vi "ForceAnnotationMan.vi"(4 "EnReturnForce":bool, 5 "EnFullAngle":bool, 6 "SpectConfig":T4, 7 "FirstTouch":T3={"FirstPeakforce"=0.2, "F_LengthView"=0, "A_LengthView "=0} {"FirstPeakforce" format="%#_13g"}, 8 "ShowName":cluster{"ShowArrow":bool, "Alias":bool}, 9 "Test Name":string(combo)="WDW", 10 "Graph Up":refnum<vi>, 11 "Graph Down":refnum<vi>) -> (0 "MaxForceUp":T2, 1 "Result Up":T1, 2 "Result Down":T1, 3 "MaxForceDown":T2)   [LabVIEW 2017]
uses:
  <vilib>/Utility/miscctls.llb/LVAnnotationListTypeDef.ctl
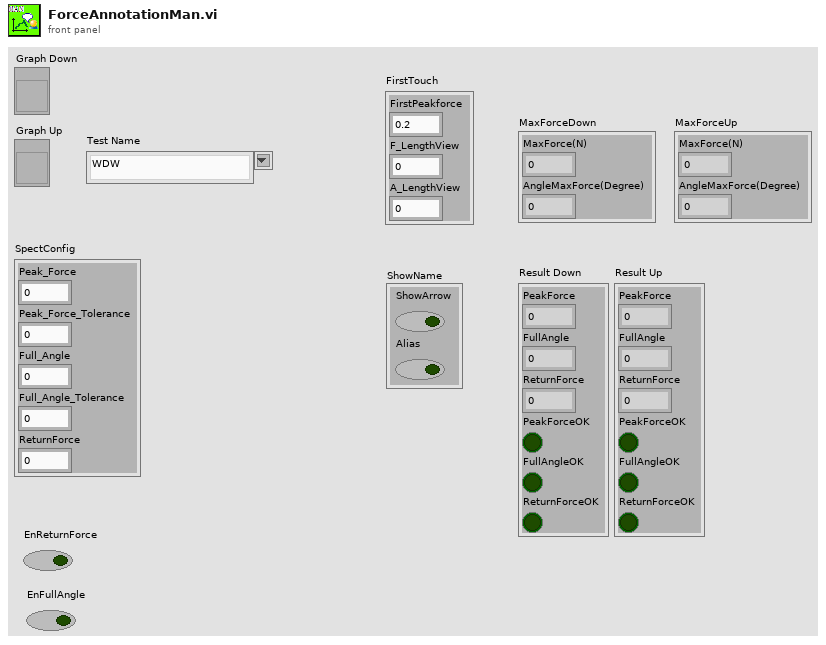
[diagram p1: front panel]
types:
  T1 = cluster{"PeakForce":dbl, "FullAngle":dbl, "ReturnForce":dbl, "PeakForceOK":bool, "FullAngleOK":bool, "ReturnForceOK":bool}
  T2 = cluster{"MaxForce(N)":dbl, "AngleMaxForce(Degree)":dbl}
  T3 = cluster{"FirstPeakforce":dbl, "F_LengthView":i32, "A_LengthView ":i32}
  T4 = cluster{"Peak_Force":dbl, "Peak_Force_Tolerance":dbl, "Full_Angle":dbl, "Full_Angle_Tolerance":dbl, "ReturnForce":dbl}
  T5 = cluster{"FirstForce":dbl, "LengthView":i32, "Name":string}
  T6 = typedef "LVAnnotationListTypeDef.ctl" = cluster{"Name":string, "Color":u32, "Style":u8, "Point Style":u8, "Name Visible":bool, "Allow Drag":bool, "Annotation Mode":u32, "Plot":i32, "Index":i32, "Position":cluster{"X":dbl, "Y":dbl}, "X Scale":u32, "Y Scale":u32, "Show Arrow":bool, "Lock Name":bool, "Plot Area":i32, "Label Offset":cluster{"X":dbl, "Y":dbl}}[]
  T7 = cluster{"Annotation List[0]":cluster{"Name":string, "Color":u32, "Style":u8, "Point Style":u8, "Name Visible":bool, "Allow Drag":bool, "Annotation Mode":u32, "Plot":i32, "Index":i32, "Position":cluster{"X":dbl, "Y":dbl}, "X Scale":u32, "Y Scale":u32, "Show Arrow":bool, "Lock Name":bool, "Plot Area":i32, "Label Offset":cluster{"X":dbl, "Y":dbl}}, "Annotation List[1]":cluster{"Name":string, "Color":u32, "Style":u8, "Point Style":u8, "Name Visible":bool, "Allow Drag":bool, "Annotation Mode":u32, "Plot":i32, "Index":i32, "Position":cluster{"X":dbl, "Y":dbl}, "X Scale":u32, "Y Scale":u32, "Show Arrow":bool, "Lock Name":bool, "Plot Area":i32, "Label Offset":cluster{"X":dbl, "Y":dbl}}, "Annotation List[2]":cluster{"Name":string, "Color":u32, "Style":u8, "Point Style":u8, "Name Visible":bool, "Allow Drag":bool, "Annotation Mode":u32, "Plot":i32, "Index":i32, "Position":cluster{"X":dbl, "Y":dbl}, "X Scale":u32, "Y Scale":u32, "Show Arrow":bool, "Lock Name":bool, "Plot Area":i32, "Label Offset":cluster{"X":dbl, "Y":dbl}}, "Annotation List[3]":cluster{"Name":string, "Color":u32, "Style":u8, "Point Style":u8, "Name Visible":bool, "Allow Drag":bool, "Annotation Mode":u32, "Plot":i32, "Index":i32, "Position":cluster{"X":dbl, "Y":dbl}, "X Scale":u32, "Y Scale":u32, "Show Arrow":bool, "Lock Name":bool, "Plot Area":i32, "Label Offset":cluster{"X":dbl, "Y":dbl}}, "Annotation List[4]":cluster{"Name":string, "Color":u32, "Style":u8, "Point Style":u8, "Name Visible":bool, "Allow Drag":bool, "Annotation Mode":u32, "Plot":i32, "Index":i32, "Position":cluster{"X":dbl, "Y":dbl}, "X Scale":u32, "Y Scale":u32, "Show Arrow":bool, "Lock Name":bool, "Plot Area":i32, "Label Offset":cluster{"X":dbl, "Y":dbl}}, "Annotation List[5]":cluster{"Name":string, "Color":u32, "Style":u8, "Point Style":u8, "Name Visible":bool, "Allow Drag":bool, "Annotation Mode":u32, "Plot":i32, "Index":i32, "Position":cluster{"X":dbl, "Y":dbl}, "X Scale":u32, "Y Scale":u32, "Show Arrow":bool, "Lock Name":bool, "Plot Area":i32, "Label Offset":cluster{"X":dbl, "Y":dbl}}, "Annotation List[6]":cluster{"Name":string, "Color":u32, "Style":u8, "Point Style":u8, "Name Visible":bool, "Allow Drag":bool, "Annotation Mode":u32, "Plot":i32, "Index":i32, "Position":cluster{"X":dbl, "Y":dbl}, "X Scale":u32, "Y Scale":u32, "Show Arrow":bool, "Lock Name":bool, "Plot Area":i32, "Label Offset":cluster{"X":dbl, "Y":dbl}}, "Annotation List[7]":cluster{"Name":string, "Color":u32, "Style":u8, "Point Style":u8, "Name Visible":bool, "Allow Drag":bool, "Annotation Mode":u32, "Plot":i32, "Index":i32, "Position":cluster{"X":dbl, "Y":dbl}, "X Scale":u32, "Y Scale":u32, "Show Arrow":bool, "Lock Name":bool, "Plot Area":i32, "Label Offset":cluster{"X":dbl, "Y":dbl}}, "Annotation List[8]":cluster{"Name":string, "Color":u32, "Style":u8, "Point Style":u8, "Name Visible":bool, "Allow Drag":bool, "Annotation Mode":u32, "Plot":i32, "Index":i32, "Position":cluster{"X":dbl, "Y":dbl}, "X Scale":u32, "Y Scale":u32, "Show Arrow":bool, "Lock Name":bool, "Plot Area":i32, "Label Offset":cluster{"X":dbl, "Y":dbl}}}
  T8 = cluster{"Name":string, "Color":u32, "Style":u8, "Point Style":u8, "Name Visible":bool, "Allow Drag":bool, "Annotation Mode":u32, "Plot":i32, "Index":i32, "Position":cluster{"X":dbl, "Y":dbl}, "X Scale":u32, "Y Scale":u32, "Show Arrow":bool, "Lock Name":bool, "Plot Area":i32, "Label Offset":cluster{"X":dbl, "Y":dbl}}[]
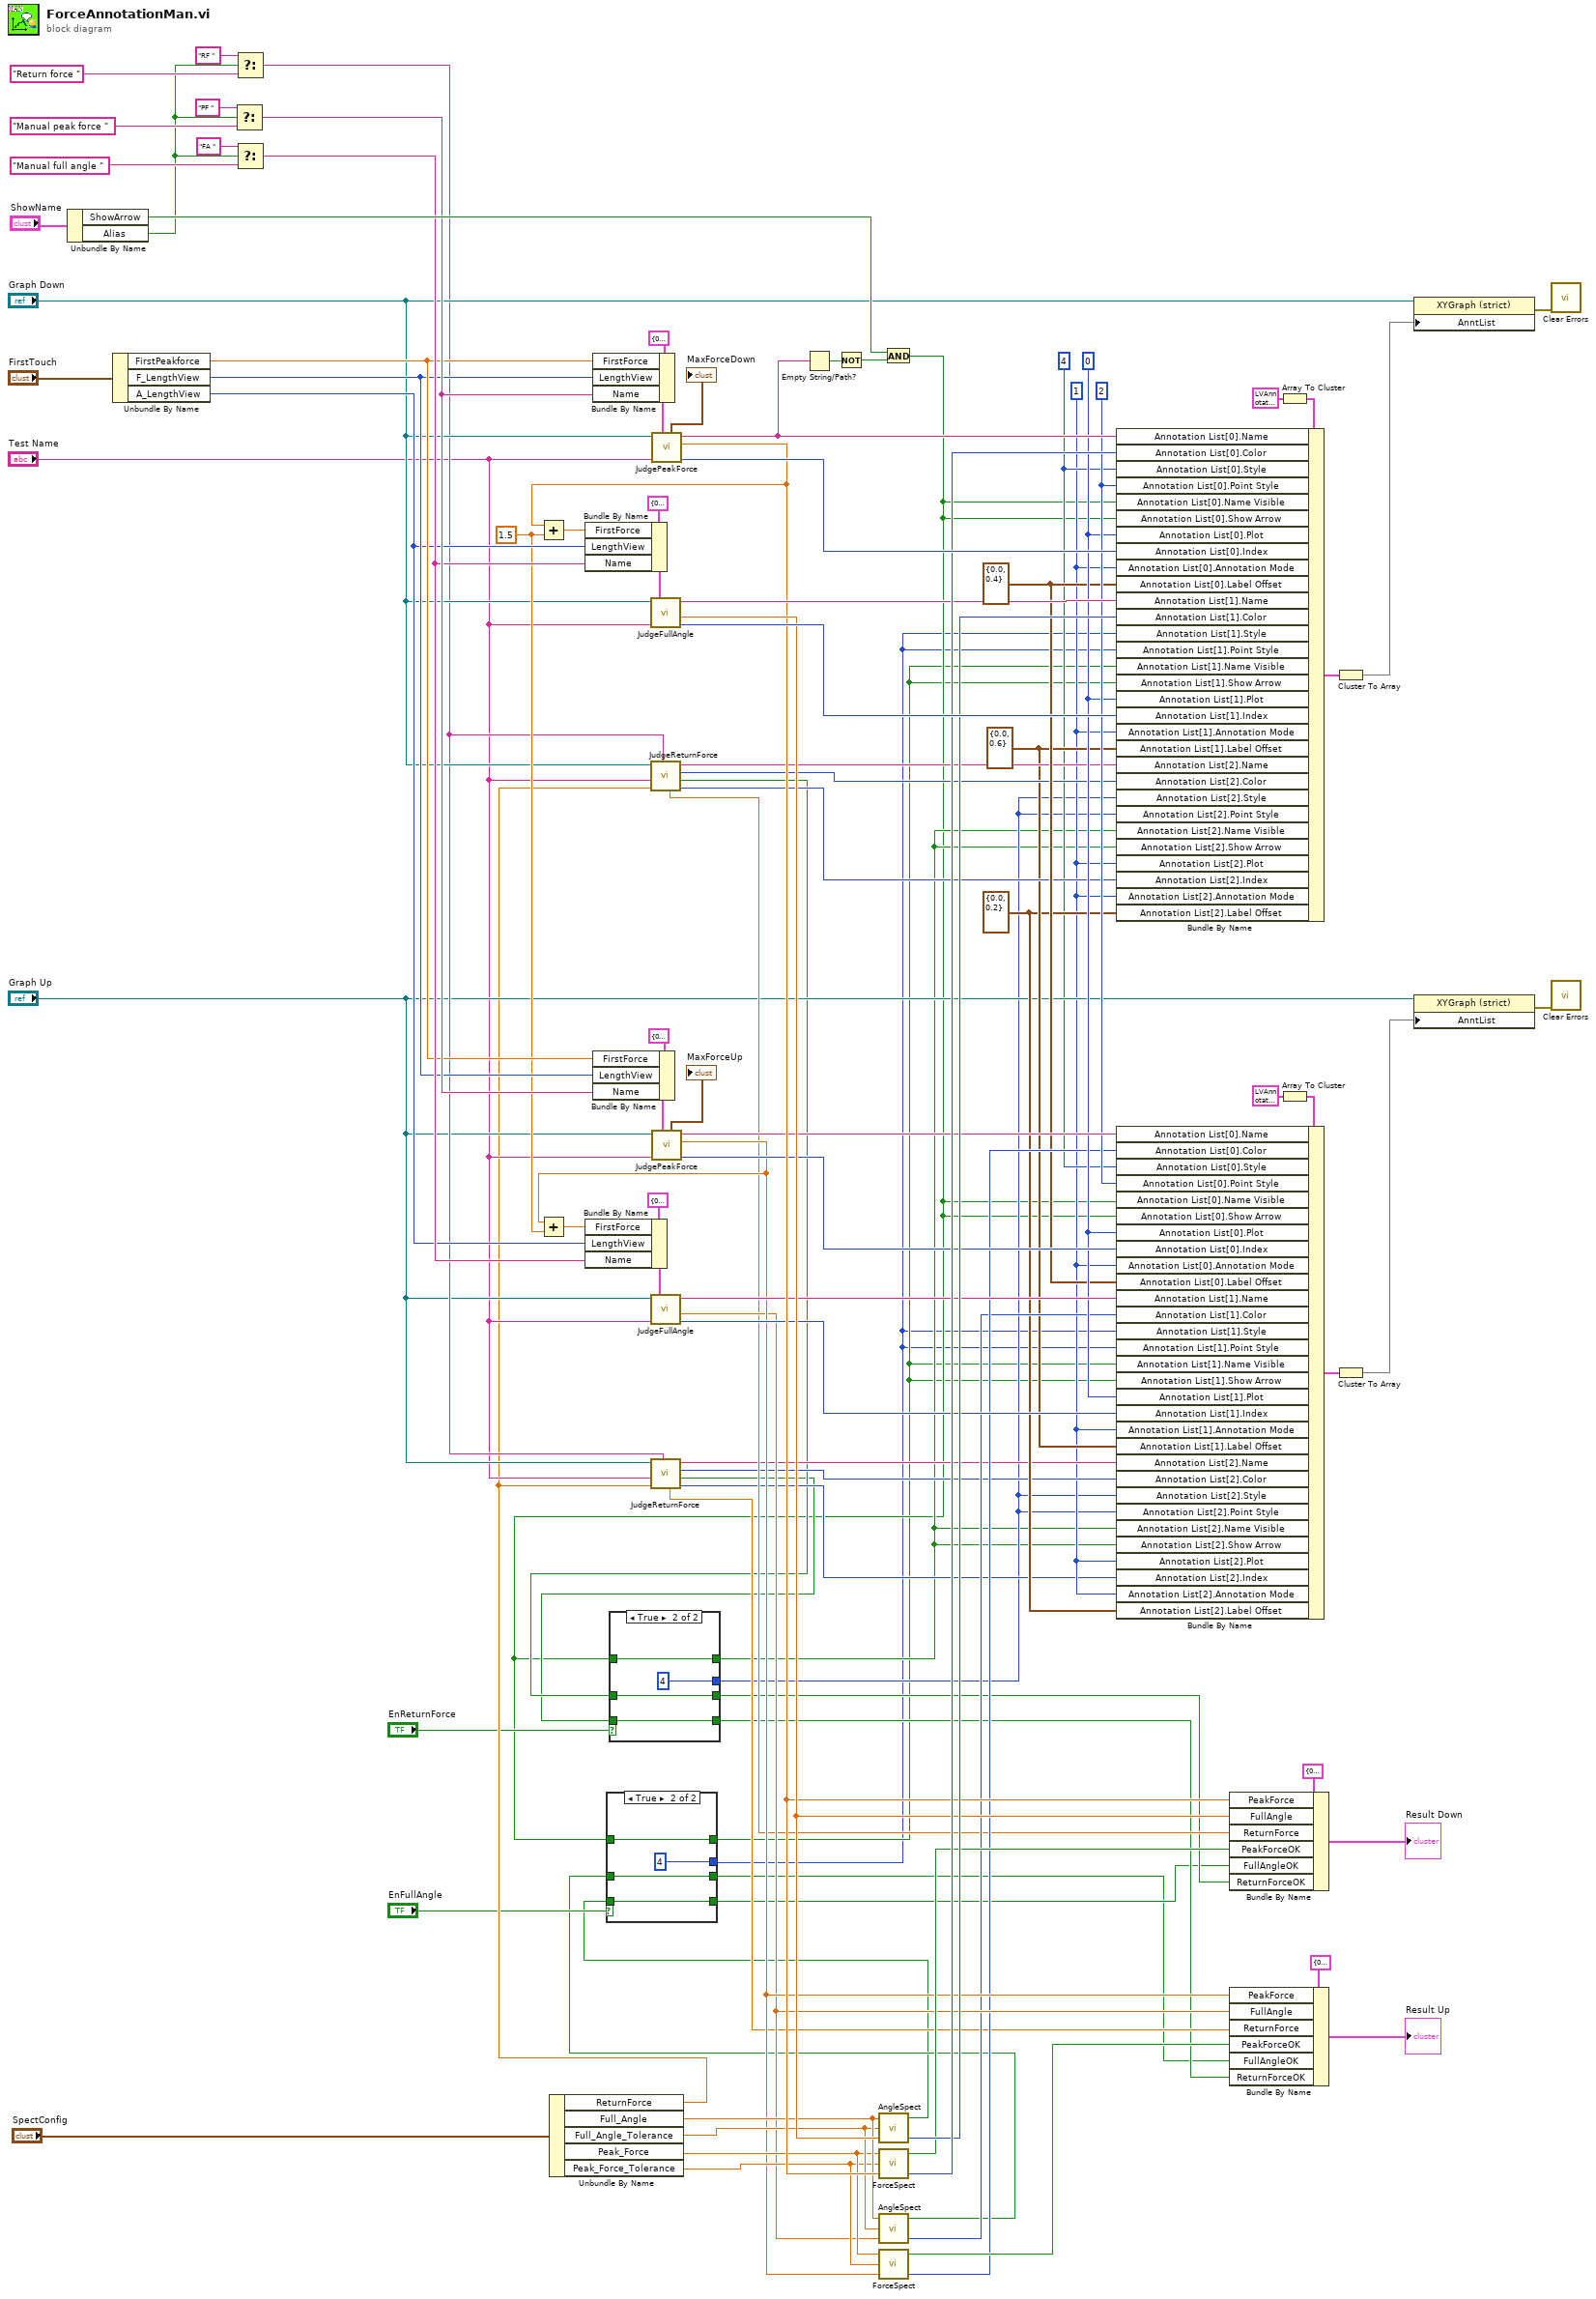
[diagram p0: block diagram]
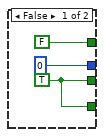
[diagram p2: hidden frame]
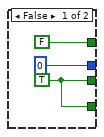
[diagram p3: hidden frame]
diagram:
  w26 = cluster{"X":dbl, "Y":dbl} {"X"=0.0, "Y"=0.2} ("Annotation List[2].Label Offset")
  w42 = 0 ("Annotation List[0].Plot")
  w38 = 1.5 ("y")
  w43 = u8 2 ("Annotation List[0].Point Style")
  w27 = cluster{"X":dbl, "Y":dbl} {"X"=0.0, "Y"=0.6} ("Annotation List[2].Label Offset")
  w39 = cluster{"X":dbl, "Y":dbl} {"X"=0.0, "Y"=0.4} ("Annotation List[0].Label Offset")
  w18 = u32 1 ("Annotation List[0].Annotation Mode")
  w19 = u8 4 ("Annotation List[0].Style")
  n1 = Unbundle By Name("ShowName") -> ("ShowArrow"=w88:bool, "Alias"=w34:bool)
  n2 = Unbundle By Name("FirstTouch") -> ("FirstPeakforce"=w58:dbl, "F_LengthView"=w57:i32, "A_LengthView"=w56:i32)
  n3 = Select(t="PF ", s=w34, f="Manual peak force " ("Name")) -> (s? t:f=w60:string)
  n4 = Select(t="RF ", s=w34, f="Return force " ("Name")) -> (s? t:f=w24:string)
  n5 = Select(t="FA ", s=w34, f="Manual full angle " ("Name")) -> (s? t:f=w59:string)
  n6 = Unbundle By Name("SpectConfig") -> ("ReturnForce"=w21:dbl, "Full_Angle"=w55:dbl, "Full_Angle_Tolerance"=w54:dbl, "Peak_Force"=w53:dbl, "Peak_Force_Tolerance"=w52:dbl)
  n7 = Bundle By Name(cluster=T5 {"FirstForce"=0.18, "LengthView"=30, "Name"="Peak Force"} ("Config"), "FirstForce"=w58, "LengthView"=w57, "Name"=w60) -> (w77:T5)
  n8 = Bundle By Name(cluster=T5 {"FirstForce"=0.18, "LengthView"=30, "Name"="Peak Force"} ("Config"), "FirstForce"=w58, "LengthView"=w57, "Name"=w60) -> (w67:T5)
  n9 = call "JudgeReturnForce.vi"("Name"=w24, "ReturnForce"=w21, "Test Name"="Test Name", "GraphDown"="Graph Down") -> ("IndexOut"=w31:i32, "Result"=w12:bool, "ColorResult"=w32:u32, "ReturnForceValue"=w33:string, "ReturnForce"=w28:dbl)  [unwired: 3 in]
  n10 = call "JudgeReturnForce.vi"("Name"=w24, "ReturnForce"=w21, "Test Name"="Test Name", "GraphDown"="Graph Up") -> ("IndexOut"=w17:i32, "Result"=w10:bool, "ColorResult"=w20:u32, "ReturnForceValue"=w25:string, "ReturnForce"=w16:dbl)  [unwired: 3 in]
  n11 = call "JudgePeakForce.vi"("Config"=w77, "Test Name"="Test Name", "XYGraph"="Graph Down") -> ("IndexOut"=w100:i32, "ForceOut"=w74:dbl, "Force Value"=w84:string, "MaxForce"=→"MaxForceDown":T2)  [unwired: 4 in, 1 out]
  n12 = Add(x=w74, y=w38) -> (x+y=w73:dbl)
  n13 = Bundle By Name(cluster=T5 {"FirstForce"=0.18, "LengthView"=30, "Name"="Peak Force"} ("Config"), "FirstForce"=w73, "LengthView"=w56, "Name"=w59) -> (w75:T5)
  n14 = call "JudgeFullAngle.vi"("Config"=w75, "Test Name"="Test Name", "XYGraph"="Graph Down") -> ("IndexOut"=w95:i32, "AngleOut"=w80:dbl, "Force Value"=w85:string)  [unwired: 5 in, 1 out]
  n15 = call "JudgePeakForce.vi"("Config"=w67, "Test Name"="Test Name", "XYGraph"="Graph Up") -> ("IndexOut"=w47:i32, "ForceOut"=w45:dbl, "Force Value"=w49:string, "MaxForce"=→"MaxForceUp":T2)  [unwired: 4 in, 1 out]
  n16 = Add(x=w45, y=w38) -> (x+y=w70:dbl)
  n17 = Bundle By Name(cluster=T5 {"FirstForce"=0.18, "LengthView"=30, "Name"="Peak Force"} ("Config"), "FirstForce"=w70, "LengthView"=w56, "Name"=w59) -> (w69:T5)
  n18 = call "JudgeFullAngle.vi"("Config"=w69, "Test Name"="Test Name", "XYGraph"="Graph Up") -> ("IndexOut"=w46:i32, "AngleOut"=w44:dbl, "Force Value"=w48:string)  [unwired: 5 in, 1 out]
  n19 = Empty String/Path?(string/path=w84) -> (empty?=w102:bool)
  n20 = Not(x=w102) -> (.not. x?=w86:bool)
  n21 = call "AngleSpect.vi"("Angle In"=w80, "Angle Tolerance"=w54, "Angle  Spect"=w55) -> ("Angle Color"=w92:u32, "Angle OK"=w6:bool)  [unwired: 1 in]
  n22 = call "ForceSpect.vi"("Force Input"=w74, "Force Tolerance"=w52, "Force  Spect"=w53) -> ("Force Color"=w93:u32, "Force OK"=w79:bool)  [unwired: 1 in]
  n23 = call "AngleSpect.vi"("Angle In"=w44, "Angle Tolerance"=w54, "Angle  Spect"=w55) -> ("Angle Color"=w40:u32, "Angle OK"=w7:bool)  [unwired: 1 in]
  n24 = call "ForceSpect.vi"("Force Input"=w45, "Force Tolerance"=w52, "Force  Spect"=w53) -> ("Force Color"=w41:u32, "Force OK"=w50:bool)  [unwired: 1 in]
  n25 = And(x=w88, y=w86) -> (x .and. y?=w3:bool)
  n26 = case shown="True" "EnFullAngle" {
    tunnel: [0 4] -> w1
    tunnel: [FALSE w108] -> w2
    tunnel: w3 -> [_ w108]
    tunnel: w7 -> [_ w107]
    tunnel: [w103 w107] -> w4
    tunnel: w6 -> [_ w106]
    tunnel: [w103 w106] -> w5
    frame False {
      w103 = TRUE ("Result")
    }
    frame True {
    }
  }
  n27 = case shown="True" "EnReturnForce" {
    tunnel: [0 4] -> w15
    tunnel: [FALSE w115] -> w14
    tunnel: w3 -> [_ w115]
    tunnel: w12 -> [_ w114]
    tunnel: [w110 w114] -> w11
    tunnel: w10 -> [_ w113]
    tunnel: [w110 w113] -> w9
    frame False {
      w110 = TRUE ("Result")
    }
    frame True {
    }
  }
  n28 = Bundle By Name(cluster=T1 {"PeakForce"=0.0, "FullAngle"=0.0, "ReturnForce"=0.0, "PeakForceOK"=FALSE, "FullAngleOK"=FALSE, "ReturnForceOK"=FALSE} ("Result Down"), "PeakForce"=w74, "FullAngle"=w80, "ReturnForce"=w28, "PeakForceOK"=w79, "FullAngleOK"=w5, "ReturnForceOK"=w11) -> (→"Result Down":T1)
  n29 = Bundle By Name(cluster=T1 {"PeakForce"=0.0, "FullAngle"=0.0, "ReturnForce"=0.0, "PeakForceOK"=FALSE, "FullAngleOK"=FALSE, "ReturnForceOK"=FALSE} ("Result Down"), "PeakForce"=w45, "FullAngle"=w44, "ReturnForce"=w16, "PeakForceOK"=w50, "FullAngleOK"=w4, "ReturnForceOK"=w9) -> (→"Result Up":T1)
  n30 = Array To Cluster(array=T6 [{"Name"="", "Color"=0, "Style"=0, "Point Style"=0, "Name Visible"=FALSE, "Allow Drag"=FALSE, "Annotation Mode"=0, "Plot"=0, "Index"=0, "Position"={"X"=0.0, "Y"=0.0}, "X Scale"=0, "Y Scale"=0, "Show Arrow"=FALSE, "Lock Name"=FALSE, "Plot Area"=0, "Label Offset"={"X"=0.0, "Y"=0.0}}] ("Annotation List")) -> (cluster=w97:T7)
  n31 = Bundle By Name(cluster=w97, "Annotation List[0].Name"=w84, "Annotation List[0].Color"=w93, "Annotation List[0].Style"=w19, "Annotation List[0].Point Style"=w43, "Annotation List[0].Name Visible"=w3, "Annotation List[0].Show Arrow"=w3, "Annotation List[0].Plot"=w42, "Annotation List[0].Index"=w100, "Annotation List[0].Annotation Mode"=w18, "Annotation List[0].Label Offset"=w39, "Annotation List[1].Name"=w85, "Annotation List[1].Color"=w92, "Annotation List[1].Style"=w1, "Annotation List[1].Point Style"=w1, "Annotation List[1].Name Visible"=w2, "Annotation List[1].Show Arrow"=w2, "Annotation List[1].Plot"=w42, "Annotation List[1].Index"=w95, "Annotation List[1].Annotation Mode"=w18, "Annotation List[1].Label Offset"=w27, "Annotation List[2].Name"=w33, "Annotation List[2].Color"=w32, "Annotation List[2].Style"=w15, "Annotation List[2].Point Style"=w15, "Annotation List[2].Name Visible"=w14, "Annotation List[2].Show Arrow"=w14, "Annotation List[2].Plot"=w18, "Annotation List[2].Index"=w31, "Annotation List[2].Annotation Mode"=w18, "Annotation List[2].Label Offset"=w26) -> (w98:T7)
  n32 = Array To Cluster(array=T6 [{"Name"="", "Color"=0, "Style"=0, "Point Style"=0, "Name Visible"=FALSE, "Allow Drag"=FALSE, "Annotation Mode"=0, "Plot"=0, "Index"=0, "Position"={"X"=0.0, "Y"=0.0}, "X Scale"=0, "Y Scale"=0, "Show Arrow"=FALSE, "Lock Name"=FALSE, "Plot Area"=0, "Label Offset"={"X"=0.0, "Y"=0.0}}] ("Annotation List")) -> (cluster=w64:T7)
  n33 = Bundle By Name(cluster=w64, "Annotation List[0].Name"=w49, "Annotation List[0].Color"=w41, "Annotation List[0].Style"=w19, "Annotation List[0].Point Style"=w43, "Annotation List[0].Name Visible"=w3, "Annotation List[0].Show Arrow"=w3, "Annotation List[0].Plot"=w42, "Annotation List[0].Index"=w47, "Annotation List[0].Annotation Mode"=w18, "Annotation List[0].Label Offset"=w39, "Annotation List[1].Name"=w48, "Annotation List[1].Color"=w40, "Annotation List[1].Style"=w1, "Annotation List[1].Point Style"=w1, "Annotation List[1].Name Visible"=w2, "Annotation List[1].Show Arrow"=w2, "Annotation List[1].Plot"=w42, "Annotation List[1].Index"=w46, "Annotation List[1].Annotation Mode"=w18, "Annotation List[1].Label Offset"=w27, "Annotation List[2].Name"=w25, "Annotation List[2].Color"=w20, "Annotation List[2].Style"=w15, "Annotation List[2].Point Style"=w15, "Annotation List[2].Name Visible"=w14, "Annotation List[2].Show Arrow"=w14, "Annotation List[2].Plot"=w18, "Annotation List[2].Index"=w17, "Annotation List[2].Annotation Mode"=w18, "Annotation List[2].Label Offset"=w26) -> (w63:T7)
  n34 = Cluster To Array(cluster=w98) -> (array=w99:T8)
  n35 = Cluster To Array(cluster=w63) -> (array=w62:T8)
  n36 = property on="Property Node" class="XYGraph (strict)"(reference="Graph Down", "AnntList"=w99) -> (error out=w101:errorcluster)  [unwired: 1 in, 1 out]
  n37 = property on="Property Node" class="XYGraph (strict)"(reference="Graph Up", "AnntList"=w62) -> (error out=w61:errorcluster)  [unwired: 1 in, 1 out]
  n38 = call <vilib>:"Clear Errors.vi"("error in (no error)"=w101) -> ()  [unwired: 5 in, 2 out]
  n39 = call <vilib>:"Clear Errors.vi"("error in (no error)"=w61) -> ()  [unwired: 5 in, 2 out]
